vi "LVClass_Image get image data.vi"(0 "Image in":refnum<class "Image.lvclass">, 11 "error in (no error)":errorcluster) -> (4 "Image out":refnum<class "Image.lvclass">, 6 "Image data out":u32[][](array[numeric]), 15 "error out":errorcluster)   [LabVIEW 2020, in "Image.lvclass"]
uses:
  Image.lvclass
  Point2D.ctl
  LVClass_Image Read Image.vi
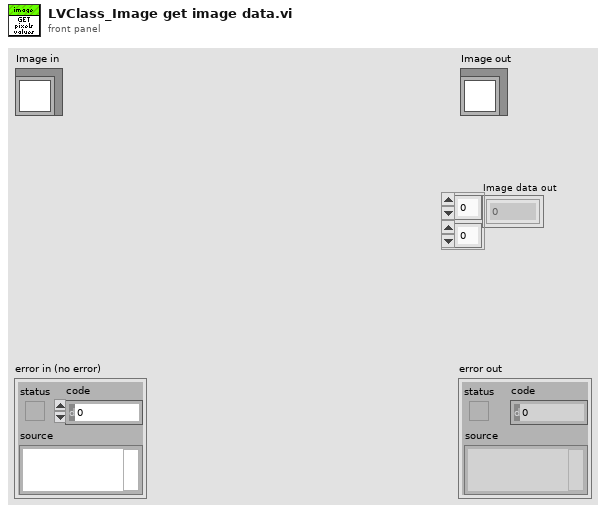
[diagram p1: front panel]
types:
  T1 = typedef "Point2D.ctl" = cluster{"X":u32, "Y":u32}
  T2 = typedef "Struct_Image.ctl" = cluster{"Image_Handler":i32, "Number of bits":T3, "ImageSize":T1}
  T3 = typedef "Data alignment enum.ctl" = enum16{"8", "16", "32"}
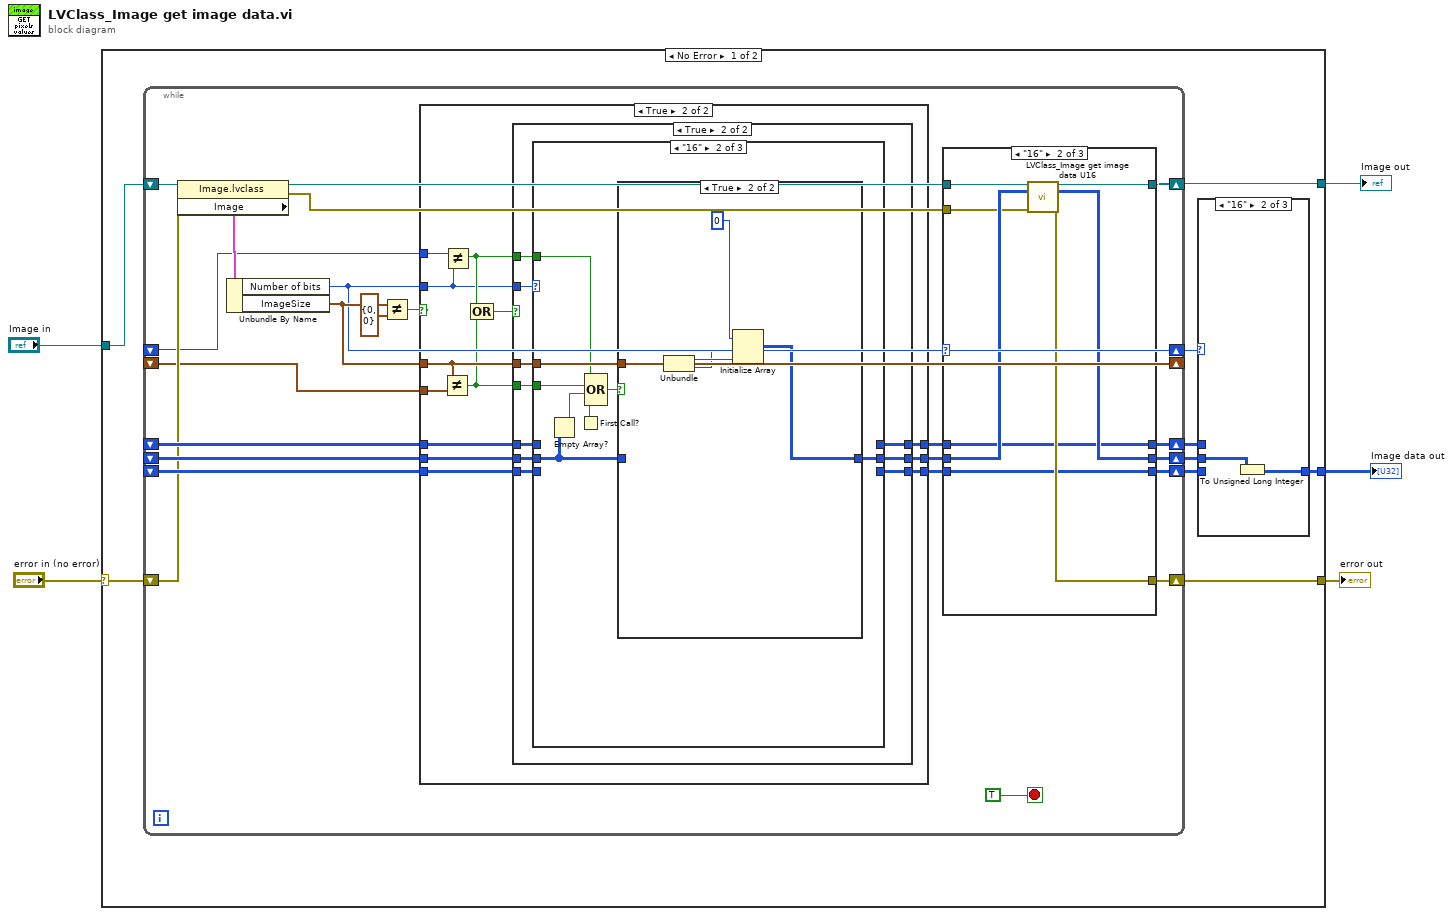
[diagram p0: block diagram]
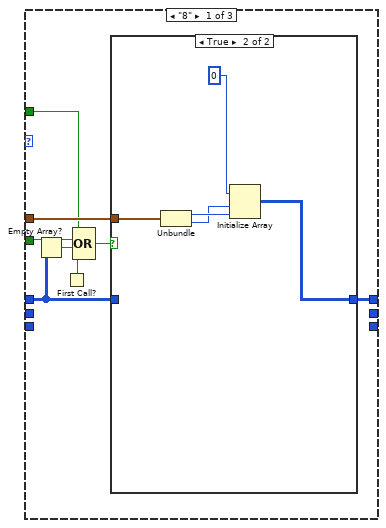
[diagram p6: hidden frame]
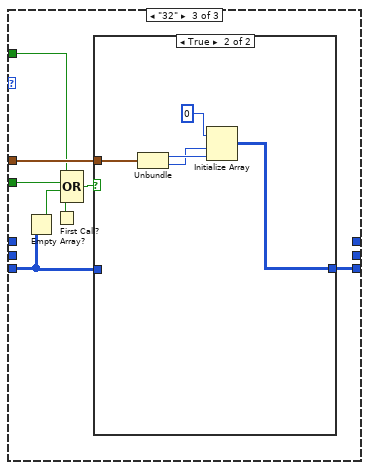
[diagram p9: hidden frame]
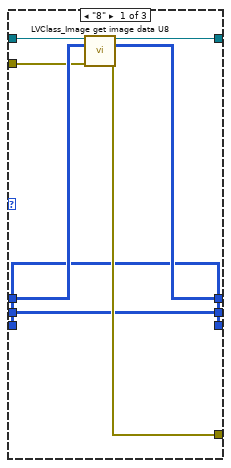
[diagram p11: hidden frame]
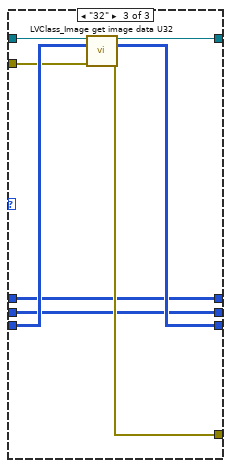
[diagram p12: hidden frame]
diagram:
  n1 = case shown="No Error" "error in (no error)" {
    selector: "error in (no error)" -> [w12 w138]
    tunnel: [w11 w138] -> w4
    tunnel: [w14 w137] -> w2
    tunnel: "Image in" -> [w13 w137]
    tunnel: [w8 _] -> w1
    frame No Error {
      n2 = while {
        shift-right: [w40] -> w9
        shift-left: _ -> [w37]
        shift-right: [w39] -> w7
        shift-left: _ -> [w36]
        shift-right: [w41] -> w6
        shift-left: _ -> [w35]
        shift-right: [w34] -> w14
        shift-left: w13 -> [w31]
        shift-right: [w33] -> w11
        shift-left: w12 -> [w30]
        shift-right: [w28] -> _
        shift-left: _ -> [w19]
        shift-right: [w20] -> w10
        shift-left: _ -> [w21]
        stop <- TRUE stop-if-true
        n3 = property class="Image.lvclass"(reference=w31, error in=w30) -> (reference out=w32:refnum<class "Image.lvclass">, error out=w26:errorcluster, "Image"=w27:T2)
        n4 = Unbundle By Name(w27) -> ("Number of bits"=w20:T3, "ImageSize"=w28:T1)
        n5 = Not Equal?(x=w28, y=T1 {"X"=0, "Y"=0}) -> (x != y?=w22:bool)
        n6 = case shown="True" w22 {
          tunnel: [w44 w57] -> w25
          tunnel: [w43 w56] -> w24
          tunnel: [w42 w55] -> w23
          tunnel: w37 -> [w44 w54]
          tunnel: w36 -> [w43 w53]
          tunnel: w35 -> [w42 w52]
          tunnel: w28 -> [_ w48]
          tunnel: w21 -> [_ w50]
          tunnel: w20 -> [_ w45]
          tunnel: w19 -> [_ w47]
          frame False {
          }
          frame True {
            n7 = Not Equal?(x=w48, y=w47) -> (x != y?=w46:bool)
            n8 = Not Equal?(x=w50, y=w45) -> (x != y?=w49:bool)
            n9 = Compound Arithmetic op=OR(w49, w46) -> (w51:bool)
            n10 = case shown="True" w51 {
              tunnel: [w60 w70] -> w57
              tunnel: [w59 w69] -> w56
              tunnel: [w58 w68] -> w55
              tunnel: w54 -> [w60 w67]
              tunnel: w53 -> [w59 w66]
              tunnel: w52 -> [w58 w65]
              tunnel: w48 -> [_ w64]
              tunnel: w45 -> [_ w63]
              tunnel: w46 -> [_ w62]
              tunnel: w49 -> [_ w61]
              frame False {
              }
              frame True {
                n11 = case shown="\"16\"" w63 {
                  tunnel: [w78 _ _] -> w70
                  tunnel: [_ w89 _] -> w69
                  tunnel: [_ _ w103] -> w68
                  tunnel: w67 -> [w73 _ _]
                  tunnel: w66 -> [_ w88 _]
                  tunnel: w65 -> [_ _ w102]
                  tunnel: w64 -> [w77 w92 w106]
                  tunnel: w62 -> [w71 w86 w100]
                  tunnel: w61 -> [w72 w87 w101]
                  frame "8" {
                    n12 = Empty Array?(array=w73) -> (empty?=w76:bool)
                    n13 = First Call?() -> (First Call?: T/F=w74:bool)
                    n14 = Compound Arithmetic op=OR(w72, w71, w76, w74) -> (w75:bool)
                    n15 = case shown="True" w75 {
                      tunnel: [w79 w84] -> w78
                      tunnel: w77 -> [_ w83]
                      tunnel: w73 -> [w79 _]
                      frame False {
                      }
                      frame True {
                        n16 = Unbundle(w83) -> ("X"=w82:u32, "Y"=w81:u32)
                        n17 = Initialize Array(u8 0 ("element"), w81, w82) -> (w84:u8[][])
                      }
                    }
                  }
                  frame "16" {
                    n18 = Empty Array?(array=w88) -> (empty?=w85:bool)
                    n19 = First Call?() -> (First Call?: T/F=w90:bool)
                    n20 = Compound Arithmetic op=OR(w87, w86, w85, w90) -> (w91:bool)
                    n21 = case shown="True" w91 {
                      tunnel: w92 -> [_ w98]
                      tunnel: [w93 w94] -> w89
                      tunnel: w88 -> [w93 _]
                      frame False {
                      }
                      frame True {
                        n22 = Unbundle(w98) -> ("X"=w97:u32, "Y"=w96:u32)
                        n23 = Initialize Array(u16 0 ("element"), w96, w97) -> (w94:u16[][])
                      }
                    }
                  }
                  frame "32" {
                    n24 = Empty Array?(array=w102) -> (empty?=w99:bool)
                    n25 = First Call?() -> (First Call?: T/F=w104:bool)
                    n26 = Compound Arithmetic op=OR(w101, w100, w99, w104) -> (w105:bool)
                    n27 = case shown="True" w105 {
                      tunnel: w106 -> [_ w112]
                      tunnel: [w107 w108] -> w103
                      tunnel: w102 -> [w107 _]
                      frame False {
                      }
                      frame True {
                        n28 = Unbundle(w112) -> ("X"=w111:u32, "Y"=w110:u32)
                        n29 = Initialize Array(u32 0 ("element"), w110, w111) -> (w108:u32[][])
                      }
                    }
                  }
                }
              }
            }
          }
        }
        n30 = case shown="\"16\"" w20 {
          tunnel: w32 -> [w116 w124 w131]
          tunnel: [w113 w121 w136] -> w41
          tunnel: [w120 w128 w135] -> w33
          tunnel: w25 -> [w119 w125 w133]
          tunnel: w24 -> [w117 w127 w132]
          tunnel: w23 -> [w113 w121 w134]
          tunnel: [w118 w125 w133] -> w40
          tunnel: [w117 w126 w132] -> w39
          tunnel: [w115 w123 w130] -> w34
          tunnel: w26 -> [w114 w122 w129]
          frame "8" {
            n31 = call "LVClass_Image get image data U8.vi"("Image in"=w116, "Image data"=w119, "error in (no error)"=w114) -> ("Image out"=w115:refnum<class "Image.lvclass">, "Image data out"=w118:u8[][], "error out"=w120:errorcluster)  [unwired: 10 in]
          }
          frame "16" {
            n32 = call "LVClass_Image get image data U16.vi"("Image in"=w124, "Image data"=w127, "error in (no error)"=w122) -> ("Image out"=w123:refnum<class "Image.lvclass">, "Image data out"=w126:u16[][], "error out"=w128:errorcluster)  [unwired: 10 in]
          }
          frame "32" {
            n33 = call "LVClass_Image get image data U32.vi"("Image in"=w131, "Image data"=w134, "error in (no error)"=w129) -> ("Image out"=w130:refnum<class "Image.lvclass">, "Image data out"=w136:u32[][], "error out"=w135:errorcluster)  [unwired: 10 in]
          }
        }
      }
      n34 = case shown="\"16\"" w10 {
        tunnel: w9 -> [w15 _ _]
        tunnel: [w15 w17 w18] -> w8
        tunnel: w7 -> [_ w16 _]
        tunnel: w6 -> [_ _ w18]
        frame "8", Default {
        }
        frame "16" {
          n35 = To Unsigned Long Integer(number=w16) -> (unsigned 32bit integer=w17:u32[][])
        }
        frame "32" {
        }
      }
    }
    frame Error {
    }
  }
  "error out" <- w4
  "Image out" <- w2
  "Image data out" <- w1
